vi "NewFolderDialogue.vi"(8 "Error In":errorcluster, 10 "Starting Name":string, 11 "AFM_Litho_Plugin.IV In":refnum<class "AFM_Litho_Plugin.IV.lvclass">) -> (0 "Error Out":errorcluster, 1 "Cancelled":bool, 2 "Name":string, 3 "AFM_Litho_Plugin.IV.lvclass Out":refnum<class "AFM_Litho_Plugin.IV.lvclass">)   [LabVIEW 2019, in "AFM_Litho_Plugin.IV.lvclass"]
uses:
  AFM_Litho_Plugin.IV.lvclass
  AFM_Litho_Plugin.IV.lvclass/AFM_Litho_Plugin.IV.ctl
panel:
  in  "Cancel":bool
  in  "OK":bool
  in  "New Folder Name":string
  # "Please enter a new folder name:"
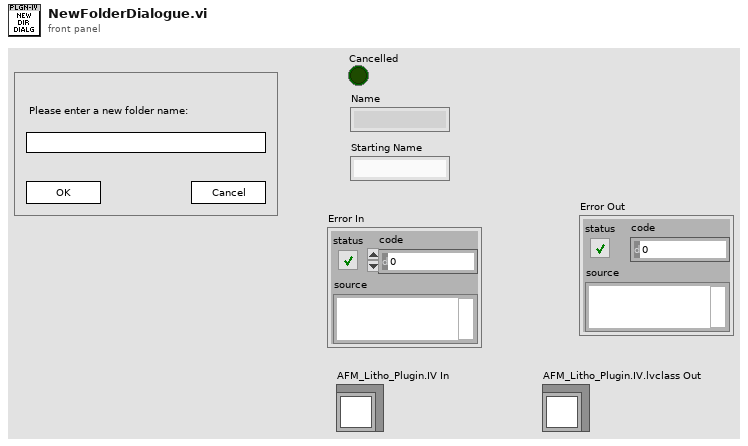
[diagram p1: front panel]
types:
  T1 = enum32{"Invalid", "Standard", "Closed", "Hidden", "Minimized", "Maximized"}
  T2 = enum32{"invalid app kind", "Development System", "Run Time System", "Student Edition", "Embedded LabVIEW", "Evaluation", "Custom"}
  T3 = cluster{"Core":cluster{"Current VI Reference":refnum<vi>, "Close Panel on Exit?":bool}, "Cancelled":bool, "Name":string, "Plugin":refnum<class "AFM_Litho_Plugin.IV.lvclass">, "BasePath":path}
  T4 = cluster{"Current VI Reference":refnum<vi>, "Close Panel on Exit?":bool}
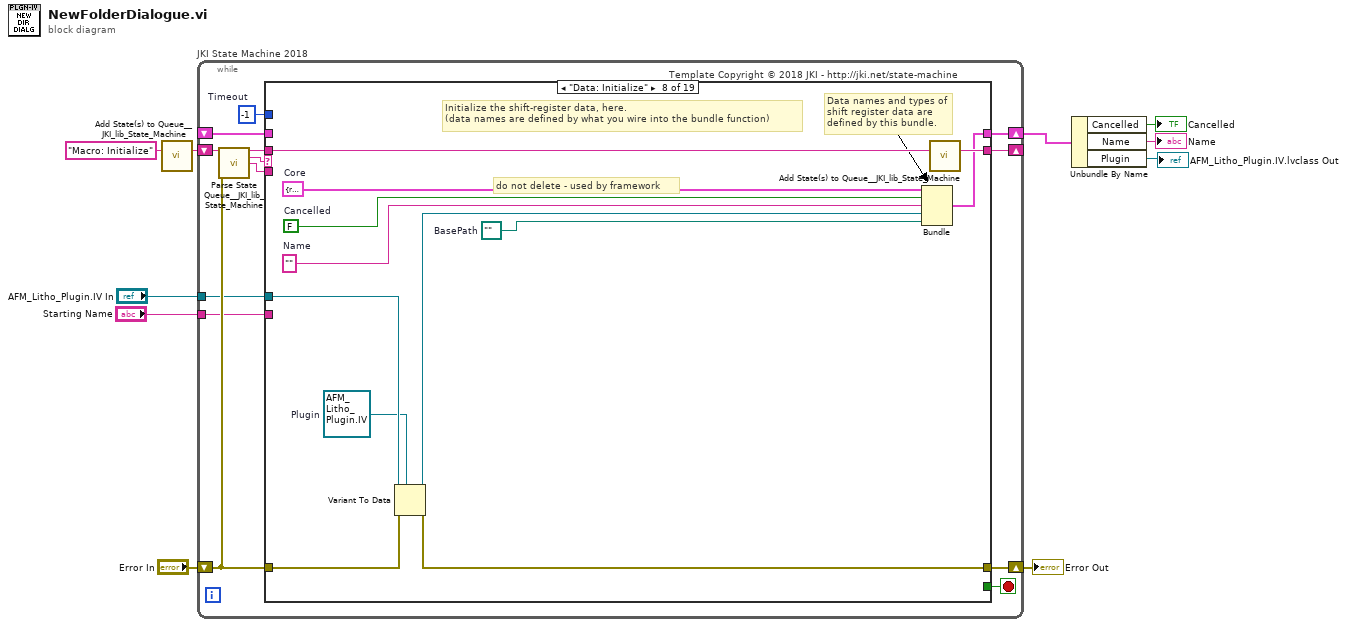
[diagram p0: block diagram]
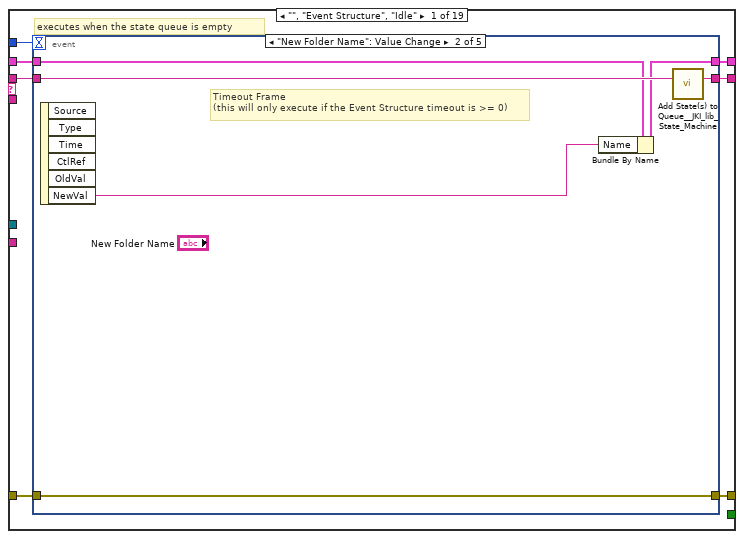
[diagram p2: hidden frame]
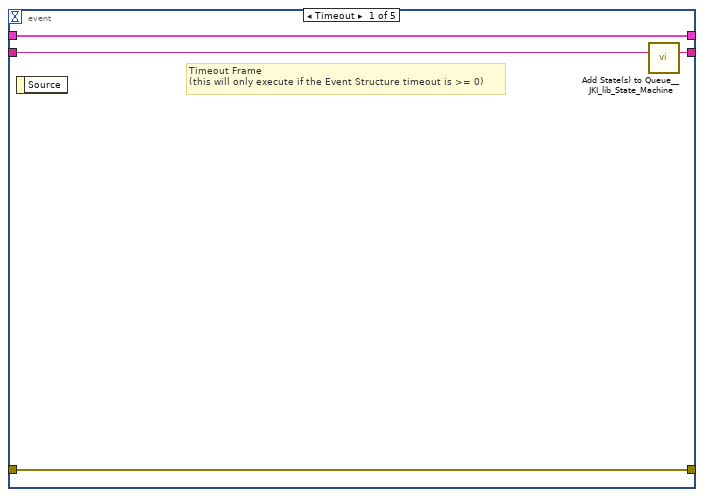
[diagram p3: hidden frame]
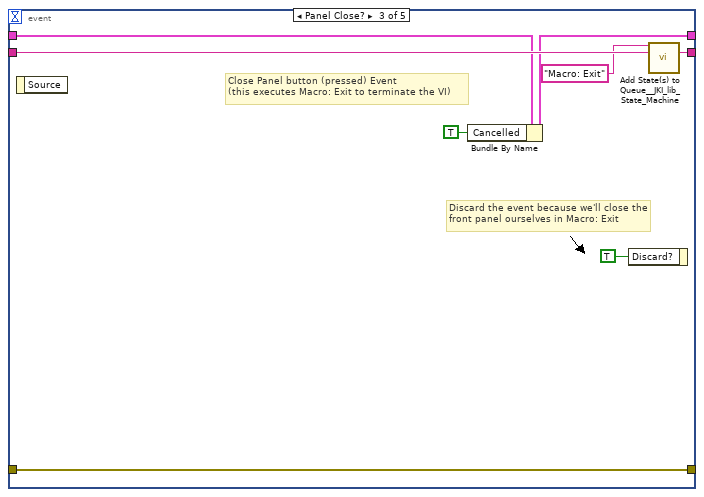
[diagram p4: hidden frame]
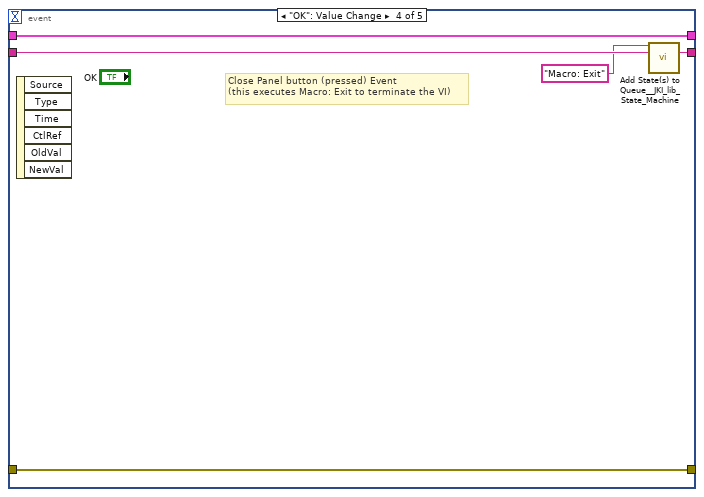
[diagram p5: hidden frame]
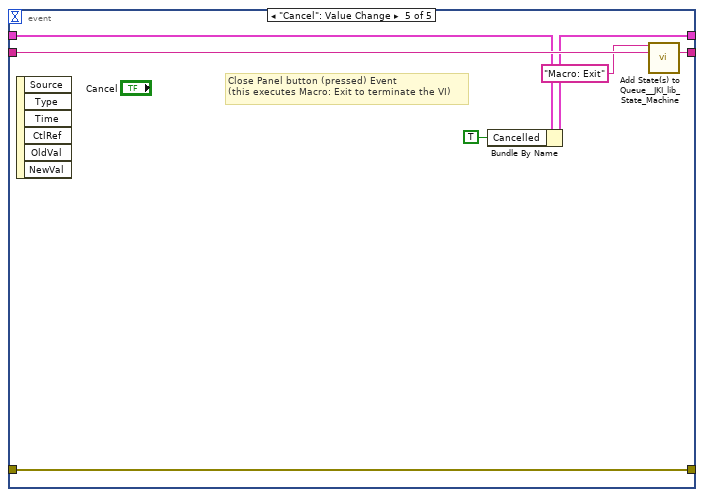
[diagram p6: hidden frame]
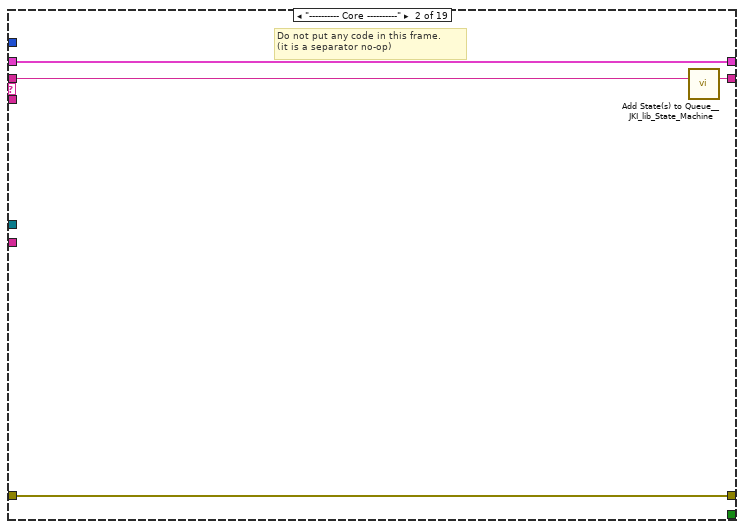
[diagram p7: hidden frame]
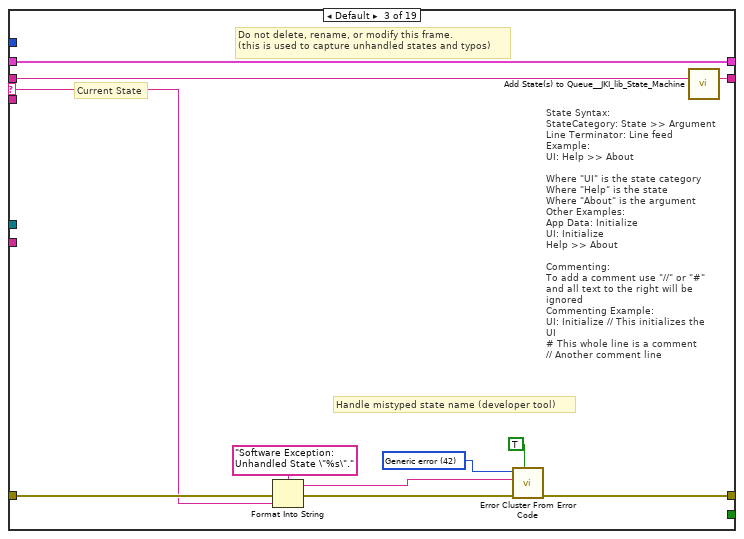
[diagram p8: hidden frame]
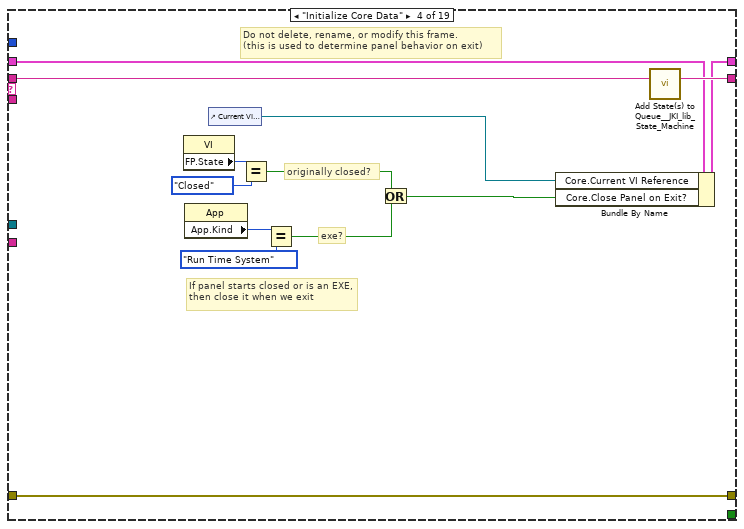
[diagram p9: hidden frame]
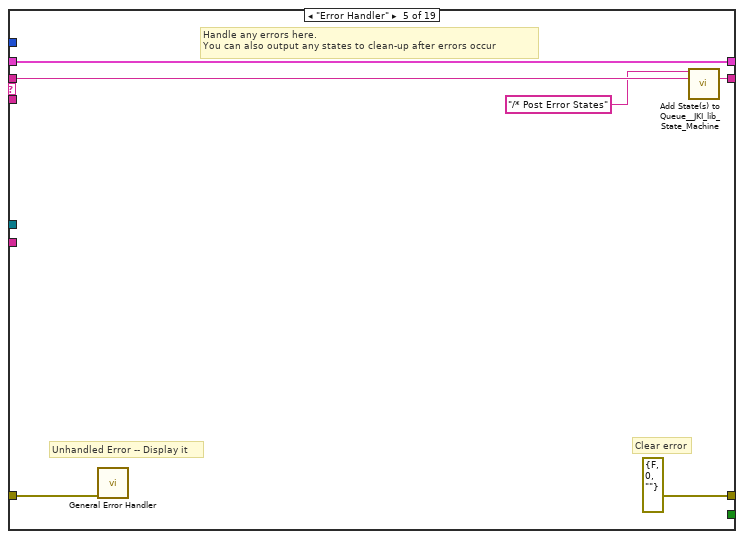
[diagram p10: hidden frame]
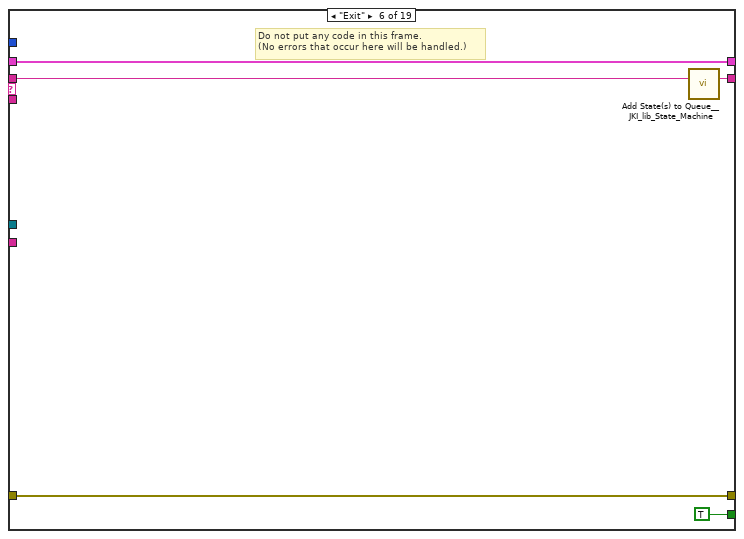
[diagram p11: hidden frame]
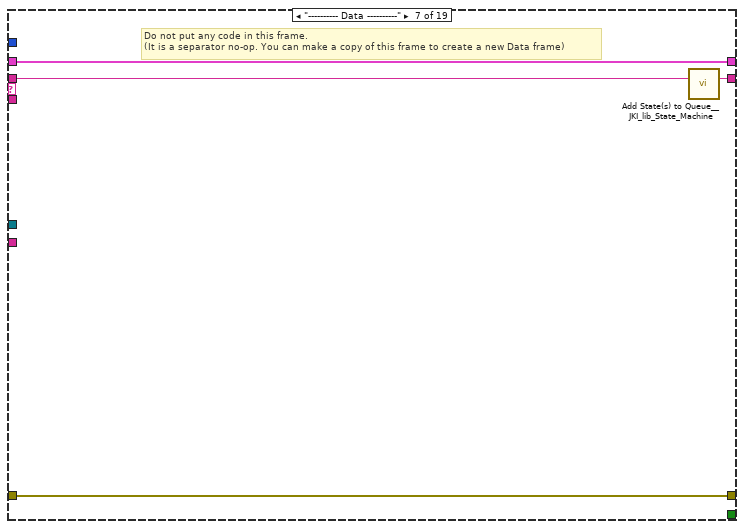
[diagram p12: hidden frame]
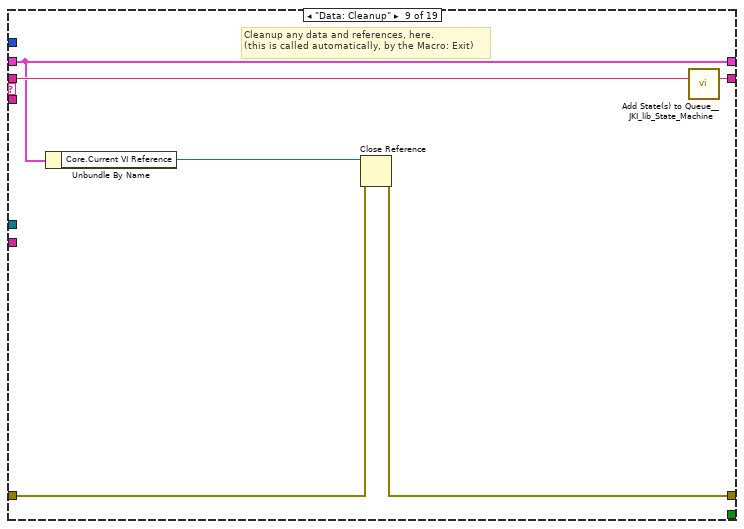
[diagram p13: hidden frame]
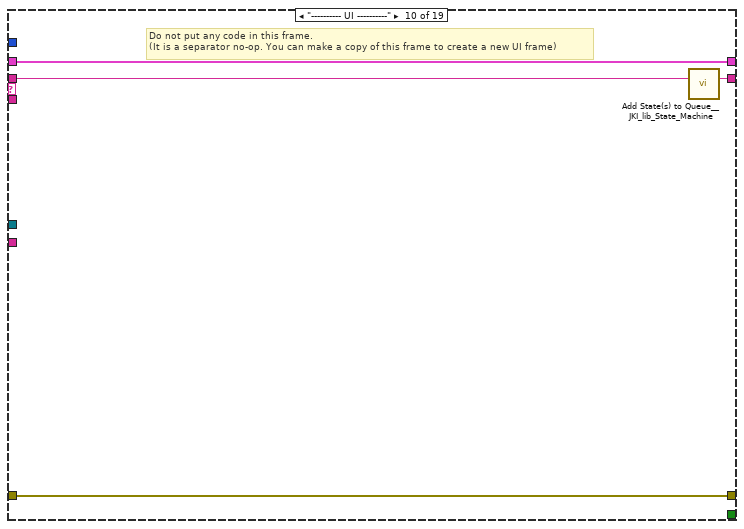
[diagram p14: hidden frame]
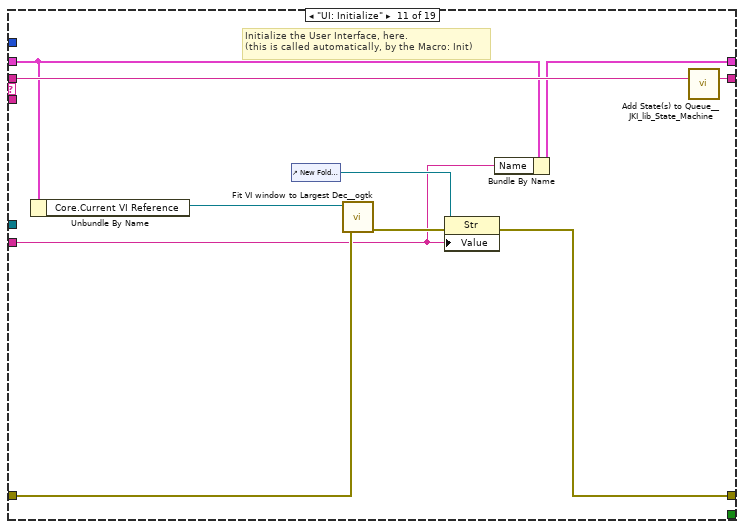
[diagram p15: hidden frame]
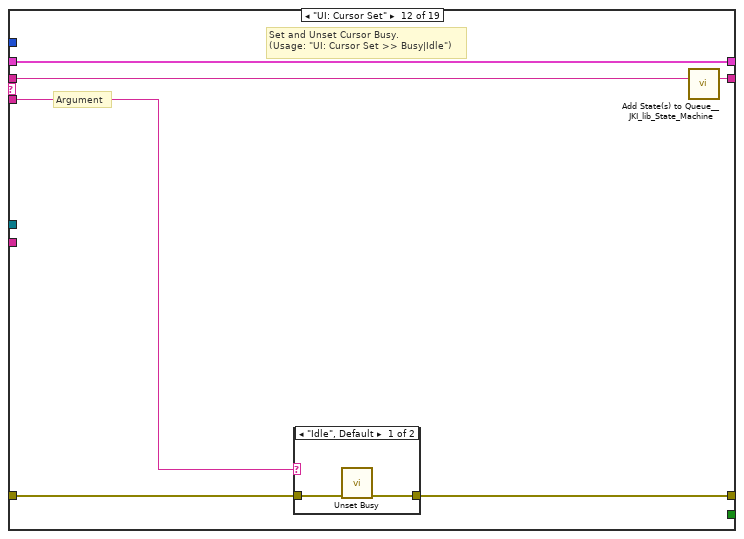
[diagram p16: hidden frame]
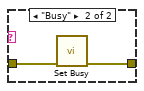
[diagram p17: hidden frame]
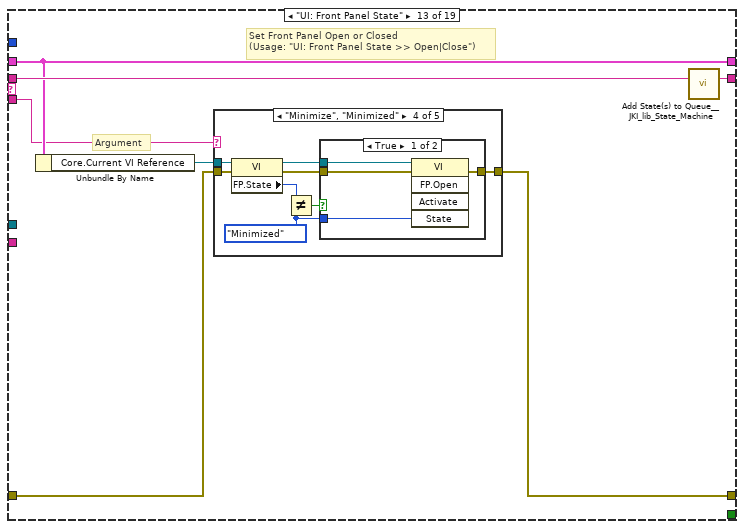
[diagram p18: hidden frame]
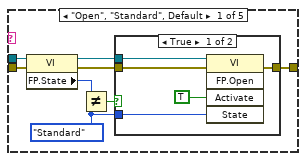
[diagram p19: hidden frame]
diagram:
  n1 = call <vilib>:"Add State(s) to Queue__JKI_lib_State_Machine.vi"("State(s) in (\"\")"="Macro: Initialize") -> ("States Out"=w10:string)  [unwired: 14 in]
  n2 = while "JKI State Machine 2018" {
    shift-right: [w16] -> w8
    shift-left: _ -> [w15]
    shift-right: [w19] -> w3
    shift-left: "Error In" -> [w13]
    shift-right: [w18] -> _
    shift-left: w10 -> [w20]
    tunnel: "Starting Name" -> [w12]
    tunnel: "AFM_Litho_Plugin.IV In" -> [w11]
    stop <- w17 stop-if-true
    w14 = -1  # Timeout
    # "Template Copyright © 2018 JKI - http://jki.net/state-machine"
    n3 = call <vilib>:"Parse State Queue__JKI_lib_State_Machine.vi"("State Queue"=w20, "Error In (no error)"=w13) -> ("Remaining States"=w22:string, "Current State"=w23:string, "Arguments"=w21:string)  [unwired: 11 in]
    n4 = case shown="\"Data: Initialize\"" w23 {
      selector: w23 -> [_ _ w65 _ _ _ _ _ _ _ _ _ _ _ _ _ _ _ _]
      tunnel: w22 -> [w30 w64 w69 w88 w94 w99 w103 w115 w121 w125 w135 w141 w152 w221 w226 w236 w240 w252 w263]
      tunnel: w21 -> [_ _ _ _ _ _ _ _ _ _ _ w136 w146 _ _ _ _ _ _]
      tunnel: w15 -> [w28 w61 w67 w81 w91 w97 w100 _ w116 w122 w126 w139 w148 w218 w223 w233 w237 w242 w256]
      tunnel: [w27 w62 w71 w85 errorcluster {"status"=FALSE, "code"=0, "source"=""} ("error out") w96 w101 w109 w117 w123 w129 w137 w149 w219 w224 w234 w238 w250 w258] -> w19
      tunnel: w13 -> [w26 w62 w70 w85 w90 w96 w101 w108 w118 w123 w131 w138 w150 w219 w224 w234 w238 w250 w258]
      tunnel: [w29 w63 w68 w87 w93 w98 w102 w114 w120 w124 w134 w140 w151 w220 w225 w235 w239 w251 w262] -> w18
      tunnel: [_ _ _ _ _ TRUE _ _ _ _ _ _ _ _ _ _ _ _ _] -> w17
      tunnel: [w25 w61 w67 w86 w91 w97 w100 w113 w116 w122 w127 w139 w148 w218 w223 w233 w237 w243 w257] -> w16
      tunnel: w14 -> [w24 _ _ _ _ _ _ _ _ _ _ _ _ _ _ _ _ _ _]
      tunnel: w12 -> [_ _ _ _ _ _ _ _ _ _ w128 _ _ _ _ _ _ w247 _]
      tunnel: w11 -> [_ _ _ _ _ _ _ w107 _ _ _ _ _ _ _ _ _ _ _]
      frame "", "Event Structure", "Idle" {
        # "executes when the state queue is empty"
        n5 = event shown="[1] \"New Folder Name\": Value Change" {
          selector: _ -> [_ _ _ _ _]
          dyn-events: _ -> [_ _ _ _ _]
          timeout: w24 -> [_ _ _ _ _]
          tunnel: w30 -> [w34 w40 w48 w53 w60]
          tunnel: [w33 w39 w47 w52 w59] -> w29
          tunnel: w28 -> [w31 w36 w42 w50 w55]
          tunnel: [w32 w38 w46 w51 w58] -> w27
          tunnel: w26 -> [w32 w38 w46 w51 w58]
          tunnel: [w31 w37 w43 w50 w56] -> w25
          event Timeout {
            # "Timeout Frame\n(this will only execute if the Event Structure timeout is >= 0)"
            n6 = event-data() -> ()  [unwired: 1 in, 1 out]
            n7 = call <vilib>:"Add State(s) to Queue__JKI_lib_State_Machine.vi"("State(s) in (\"\")"=w34) -> ("States Out"=w33:string)  [unwired: 14 in]
          }
          event "New Folder Name": Value Change {
            # "Timeout Frame\n(this will only execute if the Event Structure timeout is >= 0)"
            n8 = event-data() -> ("NewVal"=w35:string)  [unwired: 1 in, 5 out]
            n9 = Bundle By Name(cluster=w36, "Name"=w35) -> (w37:T3)
            n10 = call <vilib>:"Add State(s) to Queue__JKI_lib_State_Machine.vi"("State(s) in (\"\")"=w40) -> ("States Out"=w39:string)  [unwired: 14 in]
          }
          event Panel Close? {
            # "Discard the event because we'll close the front panel ourselves in Macro: Exit"
            # "Close Panel button (pressed) Event\n(this executes Macro: Exit to terminate the VI)"
            n11 = event-data() -> ()  [unwired: 1 in, 1 out]
            n12 = Bundle By Name(cluster=w42, "Cancelled"=TRUE) -> (w43:T3)
            n13 = event-data("Discard?"=TRUE) -> ()  [unwired: 1 in, 1 out]
            n14 = call <vilib>:"Add State(s) to Queue__JKI_lib_State_Machine.vi"("State(s) in Front (\"\")"="Macro: Exit", "State(s) in (\"\")"=w48) -> ("States Out"=w47:string)  [unwired: 13 in]
          }
          event "OK": Value Change {
            # "Close Panel button (pressed) Event\n(this executes Macro: Exit to terminate the VI)"
            n15 = event-data() -> ()  [unwired: 1 in, 6 out]
            n16 = call <vilib>:"Add State(s) to Queue__JKI_lib_State_Machine.vi"("State(s) in Front (\"\")"="Macro: Exit", "State(s) in (\"\")"=w53) -> ("States Out"=w52:string)  [unwired: 13 in]
          }
          event "Cancel": Value Change {
            # "Close Panel button (pressed) Event\n(this executes Macro: Exit to terminate the VI)"
            n17 = event-data() -> ()  [unwired: 1 in, 6 out]
            n18 = Bundle By Name(cluster=w55, "Cancelled"=TRUE) -> (w56:T3)
            n19 = call <vilib>:"Add State(s) to Queue__JKI_lib_State_Machine.vi"("State(s) in Front (\"\")"="Macro: Exit", "State(s) in (\"\")"=w60) -> ("States Out"=w59:string)  [unwired: 13 in]
          }
        }
      }
      frame "---------- Core ----------" {
        # "Do not put any code in this frame.\n(it is a separator no-op)"
        n20 = call <vilib>:"Add State(s) to Queue__JKI_lib_State_Machine.vi"("State(s) in (\"\")"=w64) -> ("States Out"=w63:string)  [unwired: 14 in]
      }
      frame Default {
        w74 = 42 items=["No error", "Argument error", "Memory is full", "Out of zone", "End of file", "File already open", "Generic file I/O error", "File not found", "File permission error", "Disk is full", "Duplicate path", "Too many files open", "System feature not enabled", "Resource file not found", "Cannot add resource", "Resource not found", "Image not found", "Image memory error", "Pen does not exist", "Config type invalid", "Config token not found", "Config parse error", "Config memory error", "Bad external code format", "Bad external code offset", "External code not present", "Null window", "Destroy window error", "Null menu", "Print aborted", "Bad print record", "Print driver error", "Windows error during printing", "Memory error during printing", "Print dialog error", "Generic print error", "Invalid device refnum", "Device not found", "Device parameter error", "Device unit error", "Cannot open device", "Device call aborted", "Generic error", "Cancelled by user", "Object ID too low", "Object ID too high", "Object not in heap", "Unknown heap", "Unknown object (invalid DefProc)", "Unknown object (DefProc not in table)", "Message out of range", "Invalid (null) method", "Unknown message", "Manager call not supported", "Bad address", "Network operation in progress", "Network operation timed out", "Connection is busy", "Network attribute not supported", "Network error", "Address in use", "System out of memory", "Connection aborted", "Connection refused", "Not connected", "Already connected", "Connection closed", "Initialization error (interapplication manager)", "Bad occurrence", "Wait on unbound occurrence handler", "Occurrence queue overflow", "Datalog type conflict", "Unused", "Unrecognized type (interapplication manager)", "Memory corrupt", "Failed to make temporary DLL", "Old CIN version", "Drag socket not found", "Failed to load drop-object", "Failed to register OLE object", "Failed to release OLE object", "Format specifier type mismatch", "Unknown format specifier", "Too few format specifiers", "Too many format specifiers", "Scan failed", "Newer CIN version", "Error converting to variant", "Runtime menu error", "Password tampered", "Variant attribute not found", "Incompatible variant data type", "Event data is not available", "Event Store is not present", "Occurrence is not found", "Event Queue is not created", "Event info is not available", "Refnum passed is NULL", "Error retrieving Class GUID", "Error retrieving CoClass GUID", "Error retrieving TypeLib GUID.", "Bad built application magic bytes.", "Specific driver is different from the specific driver associated with the Logical Name.", "There is no session opened to the class driver.", "Max Error", "MAX - Error with config objects", "MAX - Error loading configuration", "MAX - Group not supported"]
        # "State Syntax:\nStateCategory: State >> Argument\nLine Terminator: Line feed\nExample:\nUI: Help >> About\n\nWhere \"UI\" is the state category\nWhere \"Help\" is the state\nWhere \"About\" is the argument\nOther Examples:\nApp Data: Initialize\nUI: Initialize\nHelp >> About\n\nCommenting:\nTo add a comment use \"//\" or \"#\" and all text to the right will be ignored\nCommenting Example:\nUI: Initialize // This initializes the UI\n# This whole line is a comment\n// Another comment line"
        # "Current State"
        # "Do not delete, rename, or modify this frame.\n(this is used to capture unhandled states and typos)"
        # "Handle mistyped state name (developer tool)"
        n21 = Format Into String(format string="Software Exception: Unhandled State \"%s\"." ("message"), error in=w70, w65) -> (resulting string=w73:string, error out=w72:errorcluster)  [unwired: 1 in]
        n22 = call <vilib>:"Error Cluster From Error Code.vi"("show call chain? (False)"=TRUE, "error in (no error)"=w72, "error message (\"\")"=w73, "error code (0)"=w74) -> ("error out"=w71:errorcluster)  [unwired: 5 in]
        n23 = call <vilib>:"Add State(s) to Queue__JKI_lib_State_Machine.vi"("State(s) in (\"\")"=w69) -> ("States Out"=w68:string)  [unwired: 14 in]
      }
      frame "Initialize Core Data" {
        # "Do not delete, rename, or modify this frame.\n(this is used to determine panel behavior on exit)"
        # "originally closed?"
        # "exe?"
        # "If panel starts closed or is an EXE, then close it when we exit"
        n24 = property class="VI"() -> ("FP.State"=w78:T1)  [unwired: 2 in, 2 out]
        n25 = property class="App"() -> ("App.Kind"=w84:T2)  [unwired: 2 in, 2 out]
        n26 = control-ref of="Current VI Reference"() -> (w79:refnum<vi>)
        n27 = Equal?(x=w78, y=T1."Closed" ("Front Panel Window:State")) -> (x = y?=w76:bool)
        n28 = Equal?(x=w84, y=T2."Run Time System" ("Application:Kind")) -> (x = y?=w82:bool)
        n29 = Or(x=w76, y=w82) -> (x .or. y?=w80:bool)
        n30 = Bundle By Name(cluster=w81, "Core.Current VI Reference"=w79, "Core.Close Panel on Exit?"=w80) -> (w86:T3)
        n31 = call <vilib>:"Add State(s) to Queue__JKI_lib_State_Machine.vi"("State(s) in (\"\")"=w88) -> ("States Out"=w87:string)  [unwired: 14 in]
      }
      frame "Error Handler" {
        # "Unhandled Error -- Display it"
        # "Handle any errors here.\nYou can also output any states to clean-up after errors occur"
        # "Clear error"
        n32 = call <vilib>:"General Error Handler.vi"("error in (no error)"=w90) -> ()  [unwired: 10 in, 5 out]
        n33 = call <vilib>:"Add State(s) to Queue__JKI_lib_State_Machine.vi"("State(s) in Front (\"\")"="/* Post Error States", "State(s) in (\"\")"=w94) -> ("States Out"=w93:string)  [unwired: 13 in]
      }
      frame "Exit" {
        # "Do not put any code in this frame.\n(No errors that occur here will be handled.)"
        n34 = call <vilib>:"Add State(s) to Queue__JKI_lib_State_Machine.vi"("State(s) in (\"\")"=w99) -> ("States Out"=w98:string)  [unwired: 14 in]
      }
      frame "---------- Data ----------" {
        # "Do not put any code in this frame.\n(It is a separator no-op. You can make a copy of this frame to create a new Data frame)"
        n35 = call <vilib>:"Add State(s) to Queue__JKI_lib_State_Machine.vi"("State(s) in (\"\")"=w103) -> ("States Out"=w102:string)  [unwired: 14 in]
      }
      frame "Data: Initialize" {
        w104 = path ""  # BasePath
        w106 = refnum<class "AFM_Litho_Plugin.IV.lvclass"> refnum  # Plugin
        w110 = ""  # Name
        w111 = FALSE  # Cancelled
        w112 = T4 {"Current VI Reference"=refnum, "Close Panel on Exit?"=FALSE}  # Core
        # "do not delete - used by framework"
        # "Data names and types of shift register data are defined by this bundle."
        # "Initialize the shift-register data, here.\n(data names are defined by what you wire into the bundle function)"
        n36 = Variant To Data(error in=w108, type=w106, Variant=w107) -> (data=w105:refnum<class "AFM_Litho_Plugin.IV.lvclass">, error out=w109:errorcluster)
        n37 = Bundle("Core"=w112, "Cancelled"=w111, "Name"=w110, "Plugin"=w105, "BasePath"=w104) -> (w113:T3)  [unwired: 1 in]
        n38 = call <vilib>:"Add State(s) to Queue__JKI_lib_State_Machine.vi"("State(s) in (\"\")"=w115) -> ("States Out"=w114:string)  [unwired: 14 in]
      }
      frame "Data: Cleanup" {
        # "Cleanup any data and references, here.\n(this is called automatically, by the Macro: Exit)"
        n39 = Unbundle By Name(w116) -> ("Core.Current VI Reference"=w119:refnum<vi>)
        n40 = Close Reference(reference=w119, error in (no error)=w118) -> (error out=w117:errorcluster)
        n41 = call <vilib>:"Add State(s) to Queue__JKI_lib_State_Machine.vi"("State(s) in (\"\")"=w121) -> ("States Out"=w120:string)  [unwired: 14 in]
      }
      frame "---------- UI ----------" {
        # "Do not put any code in this frame.\n(It is a separator no-op. You can make a copy of this frame to create a new UI frame)"
        n42 = call <vilib>:"Add State(s) to Queue__JKI_lib_State_Machine.vi"("State(s) in (\"\")"=w125) -> ("States Out"=w124:string)  [unwired: 14 in]
      }
      frame "UI: Initialize" {
        # "Initialize the User Interface, here.\n(this is called automatically, by the Macro: Init)"
        n43 = Unbundle By Name(w126) -> ("Core.Current VI Reference"=w132:refnum<vi>)
        n44 = control-ref of="New Folder Name"() -> (w133:refnum<vi>)
        n45 = call <userlib>:"Fit VI window to Largest Dec__ogtk.vi"("error in (no error)"=w131, "VI Ref (calling VI)"=w132) -> ("error out"=w130:errorcluster)  [unwired: 4 in, 1 out]
        n46 = property class="Str"(reference=w133, error in=w130, "Value"=w128) -> (error out=w129:errorcluster)  [unwired: 1 out]
        n47 = Bundle By Name(cluster=w126, "Name"=w128) -> (w127:T3)
        n48 = call <vilib>:"Add State(s) to Queue__JKI_lib_State_Machine.vi"("State(s) in (\"\")"=w135) -> ("States Out"=w134:string)  [unwired: 14 in]
      }
      frame "UI: Cursor Set" {
        # "Argument"
        # "Set and Unset Cursor Busy.\n(Usage: \"UI: Cursor Set >> Busy|Idle\")"
        n49 = case shown="\"Idle\", Default" w136 {
          tunnel: w138 -> [w143 w145]
          tunnel: [w142 w144] -> w137
          frame "Idle", Default {
            n50 = call <vilib>:"Unset Busy.vi"("error in (no error)"=w143) -> ("error out"=w142:errorcluster)  [unwired: 10 in]
          }
          frame "Busy" {
            n51 = call <vilib>:"Set Busy.vi"("error in (no error)"=w145) -> ("error out"=w144:errorcluster)  [unwired: 9 in, 1 out]
          }
        }
        n52 = call <vilib>:"Add State(s) to Queue__JKI_lib_State_Machine.vi"("State(s) in (\"\")"=w141) -> ("States Out"=w140:string)  [unwired: 14 in]
      }
      frame "UI: Front Panel State" {
        # "Argument"
        # "Set Front Panel Open or Closed\n(Usage: \"UI: Front Panel State >> Open|Close\")"
        n53 = Unbundle By Name(w148) -> ("Core.Current VI Reference"=w147:refnum<vi>)
        n54 = case shown="\"Minimize\", \"Minimized\"" w146 {
          tunnel: w150 -> [w158 w173 w184 w197 w210]
          tunnel: [w160 w174 w186 w199 w212] -> w149
          tunnel: w147 -> [w159 w171 w185 w198 w211]
          frame "Open", "Standard", Default {
            w153 = T1."Standard" ("State")
            n55 = property class="VI"(reference=w159, error in=w158) -> (reference out=w156:refnum<vi>, error out=w157:errorcluster, "FP.State"=w155:T1)
            n56 = Not Equal?(x=w155, y=w153) -> (x != y?=w154:bool)
            n57 = case shown="True" w154 {
              tunnel: [w164 w166] -> w160
              tunnel: w157 -> [w163 w166]
              tunnel: w156 -> [w162 _]
              tunnel: w153 -> [w161 _]
              frame True {
                n58 = invoke class="VI" method="FP.Open"(reference=w162, error in=w163, "Activate"=TRUE, "State"=w161) -> (error out=w164:errorcluster)  [unwired: 1 in, 4 out]
              }
              frame False {
              }
            }
          }
          frame "Close", "Closed" {
            n59 = property class="VI"(reference=w171, error in=w173) -> (reference out=w170:refnum<vi>, error out=w172:errorcluster, "FP.State"=w168:T1)
            n60 = Not Equal?(x=w168, y=T1."Closed" ("Front Panel Window:State")) -> (x != y?=w167:bool)
            n61 = case shown="True" w167 {
              tunnel: [w175 w178] -> w174
              tunnel: w172 -> [w175 w177]
              tunnel: w170 -> [_ w176]
              frame False {
              }
              frame True {
                n62 = invoke class="VI" method="FP.Close"(reference=w176, error in=w177) -> (error out=w178:errorcluster)  [unwired: 1 in, 2 out]
              }
            }
          }
          frame "Hidden", "Hide" {
            w179 = T1."Hidden" ("State")
            n63 = property class="VI"(reference=w185, error in=w184) -> (reference out=w182:refnum<vi>, error out=w183:errorcluster, "FP.State"=w181:T1)
            n64 = Not Equal?(x=w181, y=w179) -> (x != y?=w180:bool)
            n65 = case shown="True" w180 {
              tunnel: [w190 w191] -> w186
              tunnel: w183 -> [w189 w191]
              tunnel: w182 -> [w188 _]
              tunnel: w179 -> [w187 _]
              frame True {
                n66 = invoke class="VI" method="FP.Open"(reference=w188, error in=w189, "State"=w187) -> (error out=w190:errorcluster)  [unwired: 2 in, 4 out]
              }
              frame False {
              }
            }
          }
          frame "Minimize", "Minimized" {
            w192 = T1."Minimized" ("State")
            n67 = property class="VI"(reference=w198, error in=w197) -> (reference out=w195:refnum<vi>, error out=w196:errorcluster, "FP.State"=w194:T1)
            n68 = Not Equal?(x=w194, y=w192) -> (x != y?=w193:bool)
            n69 = case shown="True" w193 {
              tunnel: [w203 w204] -> w199
              tunnel: w196 -> [w202 w204]
              tunnel: w195 -> [w201 _]
              tunnel: w192 -> [w200 _]
              frame True {
                n70 = invoke class="VI" method="FP.Open"(reference=w201, error in=w202, "State"=w200) -> (error out=w203:errorcluster)  [unwired: 2 in, 4 out]
              }
              frame False {
              }
            }
          }
          frame "Maximize", "Maximized" {
            w205 = T1."Maximized" ("State")
            n71 = property class="VI"(reference=w211, error in=w210) -> (reference out=w208:refnum<vi>, error out=w209:errorcluster, "FP.State"=w207:T1)
            n72 = Not Equal?(x=w207, y=w205) -> (x != y?=w206:bool)
            n73 = case shown="True" w206 {
              tunnel: [w216 w217] -> w212
              tunnel: w209 -> [w215 w217]
              tunnel: w208 -> [w214 _]
              tunnel: w205 -> [w213 _]
              frame True {
                n74 = invoke class="VI" method="FP.Open"(reference=w214, error in=w215, "State"=w213) -> (error out=w216:errorcluster)  [unwired: 2 in, 4 out]
              }
              frame False {
              }
            }
          }
        }
        n75 = call <vilib>:"Add State(s) to Queue__JKI_lib_State_Machine.vi"("State(s) in (\"\")"=w152) -> ("States Out"=w151:string)  [unwired: 14 in]
      }
      frame "---------- Macro ----------" {
        # "Do not put any code in this frame.\n(It is a separator no-op. You can make a copy of this frame to create a new Macro frame)"
        n76 = call <vilib>:"Add State(s) to Queue__JKI_lib_State_Machine.vi"("State(s) in (\"\")"=w221) -> ("States Out"=w220:string)  [unwired: 14 in]
      }
      frame "Macro: Initialize" {
        w222 = "Data: Initialize\nInitialize Core Data\nUI: Initialize\nPath: Base\nUI: Front Panel State >> Open"  # Data: Initialize Initialize Core Data UI: Initialize Path: Base UI: Front Panel State >> Open
        # "Initialization Macro\n(This is called once, when the VI starts)"
        n77 = call <vilib>:"Add State(s) to Queue__JKI_lib_State_Machine.vi"("State(s) in Front (\"\")"=w222, "State(s) in (\"\")"=w226) -> ("States Out"=w225:string)  [unwired: 13 in]
      }
      frame "Macro: Exit" {
        # "Exit Macro\n(This is called once, when the VI exits)"
        n78 = Unbundle By Name(w233) -> ("Core.Close Panel on Exit?"=w232:bool)
        n79 = Select(t="UI: Front Panel State >> Close", s=w232, f="") -> (s? t:f=w229:string)
        n80 = call <vilib>:"Add State(s) to Queue__JKI_lib_State_Machine.vi"("State(s) in (\"\")"=w229, "State(s) at Back (\"\")"="Path: Generate\nData: Cleanup\nExit") -> ("States Out"=w227:string)  [unwired: 13 in]
        n81 = call <vilib>:"Add State(s) to Queue__JKI_lib_State_Machine.vi"("State(s) in Front (\"\")"=w227, "State(s) in (\"\")"=w236) -> ("States Out"=w235:string)  [unwired: 13 in]
      }
      frame "---------- Path ----------" {
        # "Template Separator\n(You can make a copy of, or modify, this frame)"
        n82 = call <vilib>:"Add State(s) to Queue__JKI_lib_State_Machine.vi"("State(s) in (\"\")"=w240) -> ("States Out"=w239:string)  [unwired: 14 in]
      }
      frame "Path: Base" {
        # "Your code here.\n(You can make a copy of, or modify, this frame)"
        n83 = Unbundle By Name(w242) -> ("Plugin"=w249:refnum<class "AFM_Litho_Plugin.IV.lvclass">)
        n84 = Unbundle By Name(w249) -> ("Directory Path"=w245:path)
        n85 = Strip Path(path=w245) -> (stripped path=w244:path, name=w248:string)
        n86 = Equal?(x=w248, y=w247) -> (x = y?=w246:bool)
        n87 = Select(t=w244, s=w246, f=w245) -> (s? t:f=w241:path)
        n88 = Bundle By Name(cluster=w242, "BasePath"=w241) -> (w243:T3)
        n89 = call <vilib>:"Add State(s) to Queue__JKI_lib_State_Machine.vi"("State(s) in (\"\")"=w252) -> ("States Out"=w251:string)  [unwired: 14 in]
      }
      frame "Path: Generate" {
        # "Your code here.\n(You can make a copy of, or modify, this frame)"
        n90 = Unbundle By Name(w256) -> ("Plugin"=w254:refnum<class "AFM_Litho_Plugin.IV.lvclass">, "Cancelled"=w261:bool, "BasePath"=w260:path, "Name"=w259:string)
        n91 = case shown="False" w261 {
          tunnel: w259 -> [w271 _]
          tunnel: [w265 w280] -> w253
          tunnel: w260 -> [w272 w280]
          tunnel: w258 -> [w267 w279]
          tunnel: [w264 w279] -> _
          frame False {
            n92 = Build Path(base path=w272, name or relative path=w271) -> (appended path=w270:path)
            n93 = call <vilib>:"Check if File or Folder Exists.vi"("error in (no error)"=w267, "path"=w270) -> ("error out"=w266:errorcluster, "file or folder exists?"=w269:bool, "dup path"=w268:path)  [unwired: 7 in]
            n94 = case shown="False" w269 {
              tunnel: w268 -> [w276 w278]
              tunnel: w266 -> [w275 w277]
              tunnel: [w274 w277] -> w264
              tunnel: [w273 w278] -> w265
              frame False {
                n95 = Create Folder(path (use dialog)=w276, error in=w275) -> (created path=w273:path, error out=w274:errorcluster)  [unwired: 1 in, 1 out]
              }
              frame True {
              }
            }
          }
          frame True {
          }
        }
        n96 = Bundle By Name(cluster=w254, "Directory Path"=w253) -> (w255:refnum<class "AFM_Litho_Plugin.IV.lvclass">)
        n97 = Bundle By Name(cluster=w256, "Plugin"=w255) -> (w257:T3)
        n98 = call <vilib>:"Add State(s) to Queue__JKI_lib_State_Machine.vi"("State(s) in (\"\")"=w263) -> ("States Out"=w262:string)  [unwired: 14 in]
      }
    }
  }
  "Error Out" <- w3
  n99 = Unbundle By Name(w8) -> ("Cancelled"=→"Cancelled":bool, "Name"=→"Name":string, "Plugin"=→"AFM_Litho_Plugin.IV.lvclass Out":refnum<class "AFM_Litho_Plugin.IV.lvclass">)
